vi "Actualizar Inventario.vi"(8 "error in":errorcluster, 11 "Nombre Producto":string) -> (0 "error out":errorcluster)   [LabVIEW 2024, in "ProductControl.lvlib"]
uses:
  ProductControl.lvlib
  <vilib>/Utility/config.llb/NI_LVConfig.lvlib
  <vilib>/Utility/config.llb/Read Key (U32).vi
  <vilib>/Utility/config.llb/Write Key (U32).vi
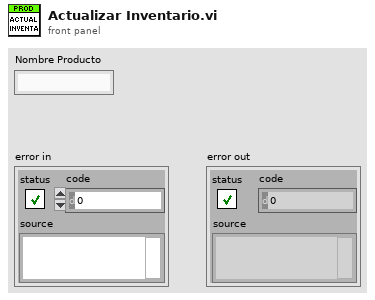
[diagram p1: front panel]
types:
  T1 = typedef "NI_LVConfig.lvlib/Config Data RefNum.ctl" = refnum<k1>
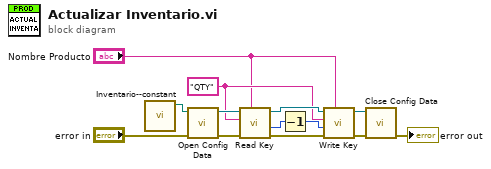
[diagram p0: block diagram]
diagram:
  w4 = "QTY" ("key")
  n1 = call "Inventario--constant.vi"() -> ("Path"=w8:path)  [unwired: 11 in]
  n2 = call <vilib>:"Open Config Data.vi"("error in (no error)"="error in", "configuration file path"=w8) -> ("error out"=w10:errorcluster, "refnum"=w6:T1)  [unwired: 7 in, 1 out]
  n3 = call-poly <vilib>:"Read Key.vi"("section"="Nombre Producto", "error in (no error)"=w10, "key"=w4, "refnum"=w6) -> ("error out"=w9:errorcluster, "value"=w3:u32, "refnum out"=w5:T1)  [unwired: 4 in, 1 out]
  n4 = Decrement(x=w3) -> (x-1=w2:u32)
  n5 = call-poly <vilib>:"Write Key.vi"("section"="Nombre Producto", "error in (no error)"=w9, "value"=w2, "key"=w4, "refnum"=w5) -> ("error out"=w13:errorcluster, "refnum out"=w7:T1)  [unwired: 4 in, 1 out]
  n6 = call <vilib>:"Close Config Data.vi"("error in (no error)"=w13, "refnum"=w7) -> ("error out"=→"error out":errorcluster)  [unwired: 8 in, 1 out]
